vi "semafinal.vi"() -> ()   [LabVIEW 2013]
panel:
  out "C":bool
  out "B":bool
  out "A":bool
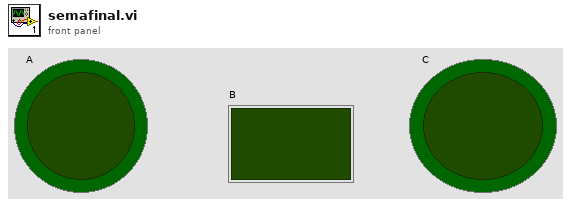
[diagram p1: front panel]
types:
  T1 = typedef "Semaphore RefNum" = refnum<k1>
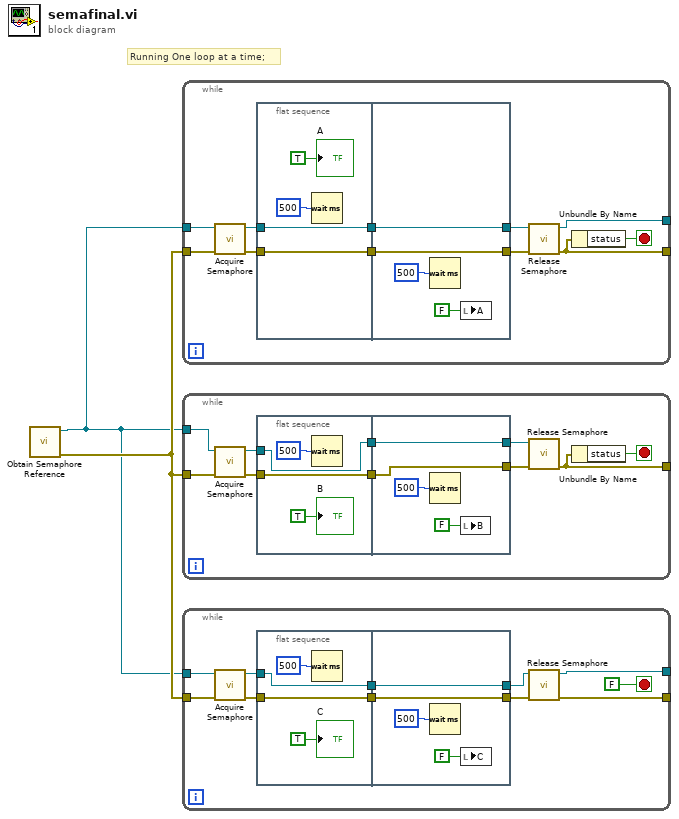
[diagram p0: block diagram]
diagram:
  # "Running One loop at a time;"
  n1 = call <vilib>:"Obtain Semaphore Reference.vi"() -> ("error out"=w2:errorcluster, "semaphore"=w1:T1)  [unwired: 5 in, 1 out]
  n2 = while {
    tunnel: w2 -> [w13]
    tunnel: [w6] -> _
    tunnel: w1 -> [w4]
    tunnel: [w3] -> _
    stop <- w5 stop-if-true
    n3 = call <vilib>:"Acquire Semaphore.vi"("error in (no error)"=w13, "semaphore"=w4) -> ("error out"=w8:errorcluster, "semaphore out"=w11:T1)  [unwired: 3 in, 1 out]
    n4 = flat-sequence {
      tunnel: [w15] -> w12
      tunnel: w11 -> [w15]
      tunnel: [w14] -> w9
      tunnel: w8 -> [w14]
      tunnel: w12 -> [w19]
      tunnel: [w19] -> w10
      tunnel: w9 -> [w18]
      tunnel: [w18] -> w7
      frame #0 {
        n5 = Wait (ms)(milliseconds to wait=u32 500) -> ()  [unwired: 1 out]
        "A" <- TRUE ("A")
      }
      frame #1 {
        n6 = Wait (ms)(milliseconds to wait=u32 500) -> ()  [unwired: 1 out]
        n7 = local write "A"(FALSE ("A")) -> ()
      }
    }
    n8 = call <vilib>:"Release Semaphore.vi"("error in (no error)"=w7, "semaphore"=w10) -> ("error out"=w6:errorcluster, "semaphore out"=w3:T1)  [unwired: 4 in]
    n9 = Unbundle By Name(w6) -> ("status"=w5:bool)
  }
  n10 = while {
    tunnel: w2 -> [w31]
    tunnel: [w24] -> _
    tunnel: w1 -> [w22]
    stop <- w23 stop-if-true
    n11 = call <vilib>:"Acquire Semaphore.vi"("error in (no error)"=w31, "semaphore"=w22) -> ("error out"=w27:errorcluster, "semaphore out"=w29:T1)  [unwired: 3 in, 1 out]
    n12 = flat-sequence {
      tunnel: [w33] -> w30
      tunnel: w29 -> [w33]
      tunnel: [w32] -> w28
      tunnel: w27 -> [w32]
      tunnel: w30 -> [w37]
      tunnel: w28 -> [w36]
      tunnel: [w37] -> w26
      tunnel: [w36] -> w25
      frame #0 {
        n13 = Wait (ms)(milliseconds to wait=u32 500) -> ()  [unwired: 1 out]
        "B" <- TRUE ("B")
      }
      frame #1 {
        n14 = Wait (ms)(milliseconds to wait=u32 500) -> ()  [unwired: 1 out]
        n15 = local write "B"(FALSE ("B")) -> ()
      }
    }
    n16 = call <vilib>:"Release Semaphore.vi"("error in (no error)"=w25, "semaphore"=w26) -> ("error out"=w24:errorcluster)  [unwired: 4 in, 1 out]
    n17 = Unbundle By Name(w24) -> ("status"=w23:bool)
  }
  n18 = while {
    tunnel: w2 -> [w50]
    tunnel: [w43] -> _
    tunnel: [w42] -> _
    tunnel: w1 -> [w41]
    stop <- FALSE stop-if-true
    n19 = call <vilib>:"Acquire Semaphore.vi"("error in (no error)"=w50, "semaphore"=w41) -> ("error out"=w46:errorcluster, "semaphore out"=w48:T1)  [unwired: 3 in, 1 out]
    n20 = flat-sequence {
      tunnel: [w52] -> w49
      tunnel: w48 -> [w52]
      tunnel: [w51] -> w47
      tunnel: w46 -> [w51]
      tunnel: w49 -> [w56]
      tunnel: w47 -> [w55]
      tunnel: [w56] -> w45
      tunnel: [w55] -> w44
      frame #0 {
        n21 = Wait (ms)(milliseconds to wait=u32 500) -> ()  [unwired: 1 out]
        "C" <- TRUE ("C")
      }
      frame #1 {
        n22 = Wait (ms)(milliseconds to wait=u32 500) -> ()  [unwired: 1 out]
        n23 = local write "C"(FALSE ("C")) -> ()
      }
    }
    n24 = call <vilib>:"Release Semaphore.vi"("error in (no error)"=w44, "semaphore"=w45) -> ("error out"=w43:errorcluster, "semaphore out"=w42:T1)  [unwired: 4 in]
  }
